vi "tester.vi"() -> ()   [LabVIEW 2013]
uses:
  Logger.lvlib
panel:
  out "error out 2":errorcluster
  in  "Channel paths":string[](array[string])
  in  "Base Log File Path":path
  out "error out":errorcluster
  out "Report Text":string
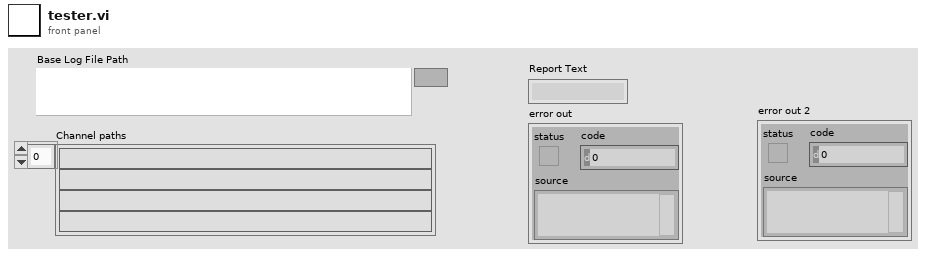
[diagram p1: front panel]
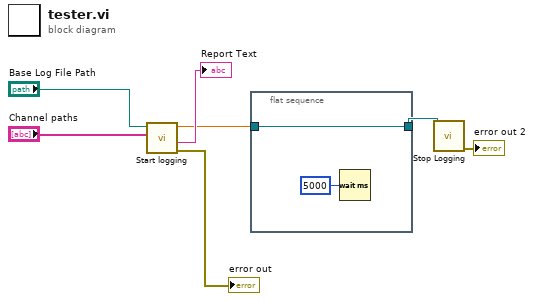
[diagram p0: block diagram]
diagram:
  n1 = call "Start logging.vi"("Channel paths"="Channel paths", "Base Log File Path"="Base Log File Path") -> ("error out"=→"error out":errorcluster, "Report Text"=→"Report Text":string, "Custom rate"=w2:dbl)  [unwired: 7 in]
  n2 = flat-sequence {
    tunnel: w2 -> [w9]
    tunnel: [w9] -> w1
    frame #0 {
      n3 = Wait (ms)(milliseconds to wait=u32 5000) -> ()  [unwired: 1 out]
    }
  }
  n4 = call "Stop Logging.vi"(11:w1) -> ("error out"=→"error out 2":errorcluster)  [unwired: 9 in, 1 out]
